vi "SubVI FM Demodulation Unwrap Phase - Continuous.vi"(1 "重置":bool, 2 "输入信号":waveform(dbl)) -> (0 "相位展开":waveform(dbl))   [LabVIEW 2015]
uses:
  <vilib>/Analysis/NI_AALPro.lvlib
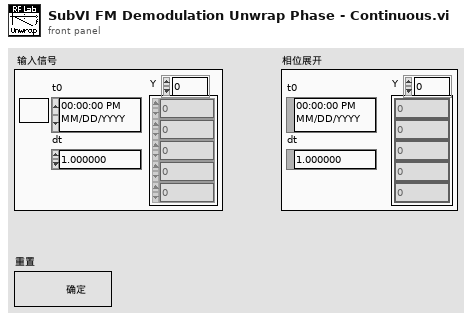
[diagram p1: front panel]
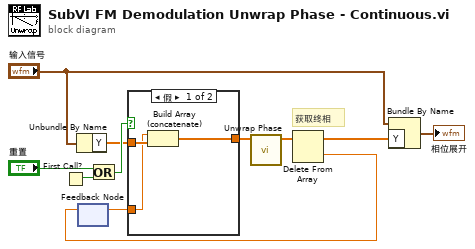
[diagram p0: block diagram]
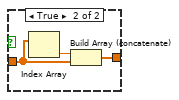
[diagram p2: hidden frame]
diagram:
  # "获取终相"
  n1 = First Call?() -> (First Call?: T/F=w11:bool)
  n2 = Unbundle By Name("输入信号") -> ("Y"=w9:dbl[])
  n3 = feedback #1() -> (w2:dbl)  [unwired: 1 in]
  n4 = Or(x="重置", y=w11) -> (x .or. y?=w10:bool)
  n5 = case shown="假" w10 {
    tunnel: w9 -> [w13 w16]
    tunnel: [w14 w15] -> w5
    tunnel: w2 -> [w12 _]
    frame False {
      n6 = Build Array (concatenate)(w12, w13) -> (w14:dbl[])
    }
    frame True {
      n7 = Index Array(array=w16) -> (element=w17:dbl)  [unwired: 1 in]
      n8 = Build Array (concatenate)(w17, w16) -> (w15:dbl[])
    }
  }
  n9 = call <vilib>:"Unwrap Phase.vi"("Phase"=w5) -> ("Unwrapped Phase"=w4:dbl[])  [unwired: 1 in, 9 out]
  n10 = Delete From Array(array=w4) -> (deleted portion=w3:dbl, array with subset deleted=w6:dbl[])  [unwired: 2 in]
  n11 = feedback-in #1(w3) -> ()
  n12 = Bundle By Name(cluster="输入信号", "Y"=w6) -> (→"相位展开":waveform(dbl))
